vi "DATEANDTIME(SubVI).vi"() -> (2 "TIME":string, 3 "DATE":string)   [LabVIEW 2020]
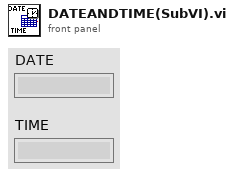
[diagram p1: front panel]
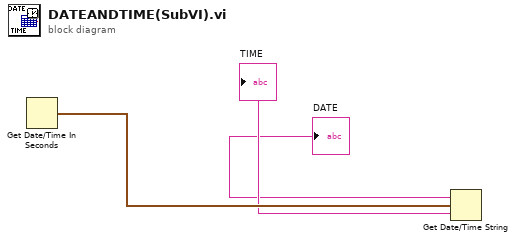
[diagram p0: block diagram]
diagram:
  n1 = Get Date/Time In Seconds() -> (seconds since 1Jan1904=w3:timestamp)
  n2 = Get Date/Time String(seconds (now)=w3) -> (date string=→"DATE":string, time string=→"TIME":string)  [unwired: 2 in]
